vi "LAb7_MSK1.vi"() -> ()   [LabVIEW 2019]
uses:
  <vilib>/addons/Modulation/Digital/General/MT Generate Bits (Galois, PN Order).vi
  <vilib>/addons/Modulation/Analog/support/mod_Set Error Source.vi
  <vilib>/addons/Modulation/Digital/Support/Common/Validators/mod_Generate Bits Validate.vi
  <vilib>/addons/Modulation/Digital/Support/Common/Validators/mod_AWGN Validate.vi
  <vilib>/addons/Modulation/Digital/Impairments/subVIs/mod_createSeeds.vi
  <vilib>/addons/Modulation/Digital/Support/Common/Validators/mod_Validate Samples Per Symbol.vi
  <vilib>/addons/Modulation/Analog/support/Validators/mod_Validate Complex Waveform.vi
  <vilib>/addons/Modulation/Analog/support/Validators/mod_WFErrorHandler.vi
  <vilib>/addons/Modulation/Digital/General/subVIs/mod_Generate Bits PN Sequence.vi
  <vilib>/addons/Modulation/Digital/Support/Common/Validators/mod_Generate Filter Coefficients Validate.vi
  <vilib>/addons/Modulation/Digital/General/subVIs/mod_Generate Filter Coefficients.vi
  <vilib>/addons/Modulation/Digital/General/MT Generate MSK System Parameters.vi
  <vilib>/addons/Modulation/Digital/General/MT Map Bits to MSK symbols.vi
  <vilib>/addons/Modulation/Digital/General/MT Apply Pulse Shaping Filter (MSK).vi
  <vilib>/Analysis/1siggen.llb/Gaussian White Noise (obs 90).vi
  <vilib>/addons/Modulation/Analog/MT Upconvert Baseband (Real).vi
  <vilib>/express/express analysis/Spectral/Block/exnSpectralBlock spectral measurements RMS poly.vi
  <vilib>/express/express analysis/Spectral/Block/exnSpectralBlock spectral measurements RMS DDT.vi
  <vilib>/addons/Modulation/Digital/General/MT Apply Matched Filter (MSK).vi
  <vilib>/addons/Modulation/Digital/General/MT Align To Ideal Symbols (MSK).vi
  <vilib>/addons/Modulation/Digital/General/MT Map MSK Symbols to Bits.vi
  <vilib>/addons/Modulation/Digital/Demodulation/MT Calculate BER After Trigger (Fibonacci PN Sequence).vi
  <vilib>/express/express analysis/Spectral/XNode/ExpressSpectralMeasurementsBlockNode.xnode
  <vilib>/addons/Modulation/niDMT.lvlib
  <vilib>/addons/Modulation/niAMT.lvlib
panel:
  in  "Differential Encoding":u16(ring)=1 items=["disable", "enable"]
  in  "Pulse Shaping Filter":u16(ring) items=["none", "Raised Cosine", "Root Raised Cos", "Gaussian"]
  out "Constellation Graph":T1(graph)
  out "Recovered Message Bits":i8[](array[numeric])
  in  "Eb/N0 (dB)":dbl=10.0 format="%.2f"
  in  "autoscale":bool
  out "BER":dbl format="%.4f"
  out "error out":errorcluster
  out "Spectrum(FFT)":dynamicdata(graph)
  in  "stop":bool
  in  "Reset":bool=TRUE
  in  "Symbol Rate(HZ)":dbl=10.0 format="%.2p"
  in  "MSK Symbols":i32
  # "MSK"
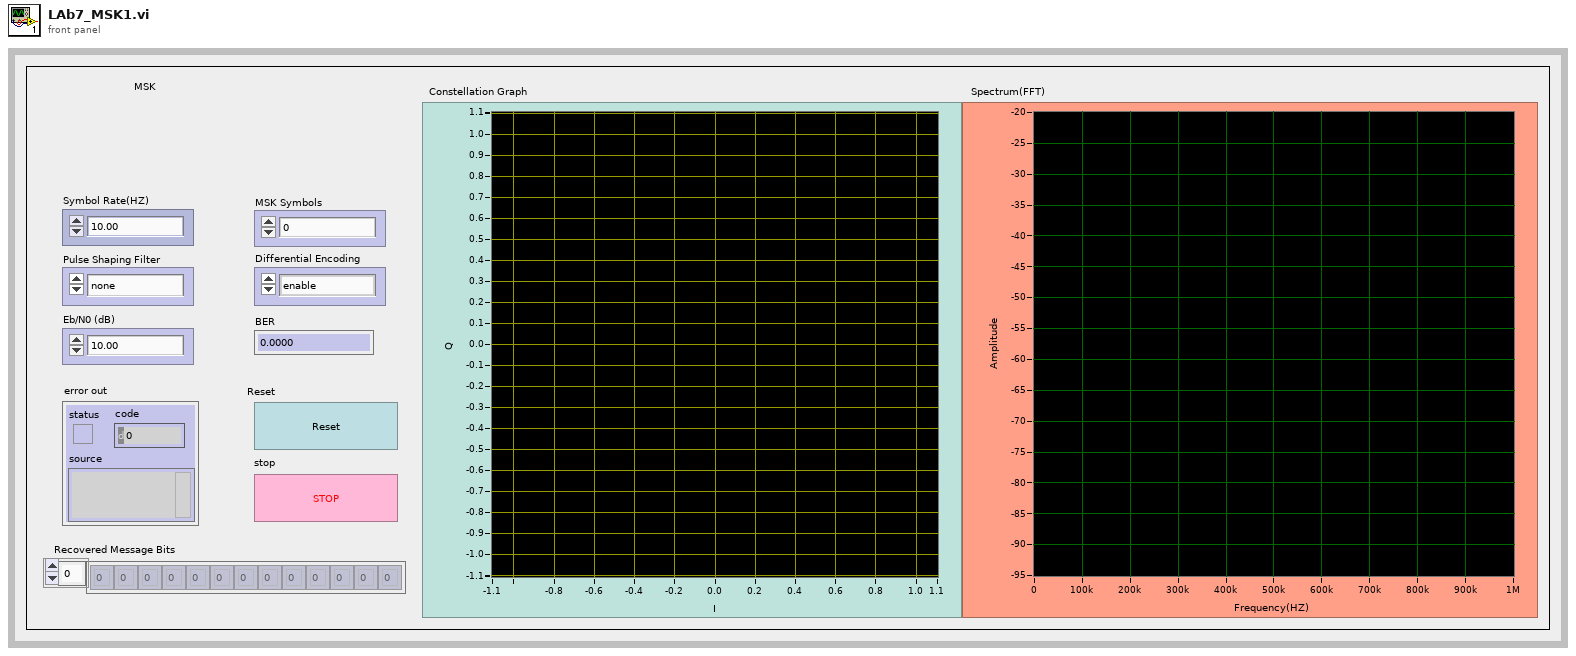
[diagram p1: front panel]
types:
  T1 = cluster{"Decimated Array":dbl[], "Decimated Array":dbl[]}[]
  T2 = enum16{"FSK", "PSK", "QAM", "MSK", "PAM", "ASK", "CPM"}
  T3 = cluster{"averaging mode":u16, "weighting mode":u16, "number of averages":u32}
  T4 = cluster{"dB On (F)":bool, "unwrap phase (F)":bool, "convert to degree (F)":bool}
  T5 = cluster{"differential encoding enable":enum16{"disable", "enable"}, "samples per symbol (16)":i32}
  T6 = typedef "niAMT.lvlib/Complex Data Waveform.ctl" = cluster{"t0":dbl, "dt":dbl, "Y":cdb[]}
  T7 = cluster{"constellation":dbl[], "oversampled data":dbl[]}[]
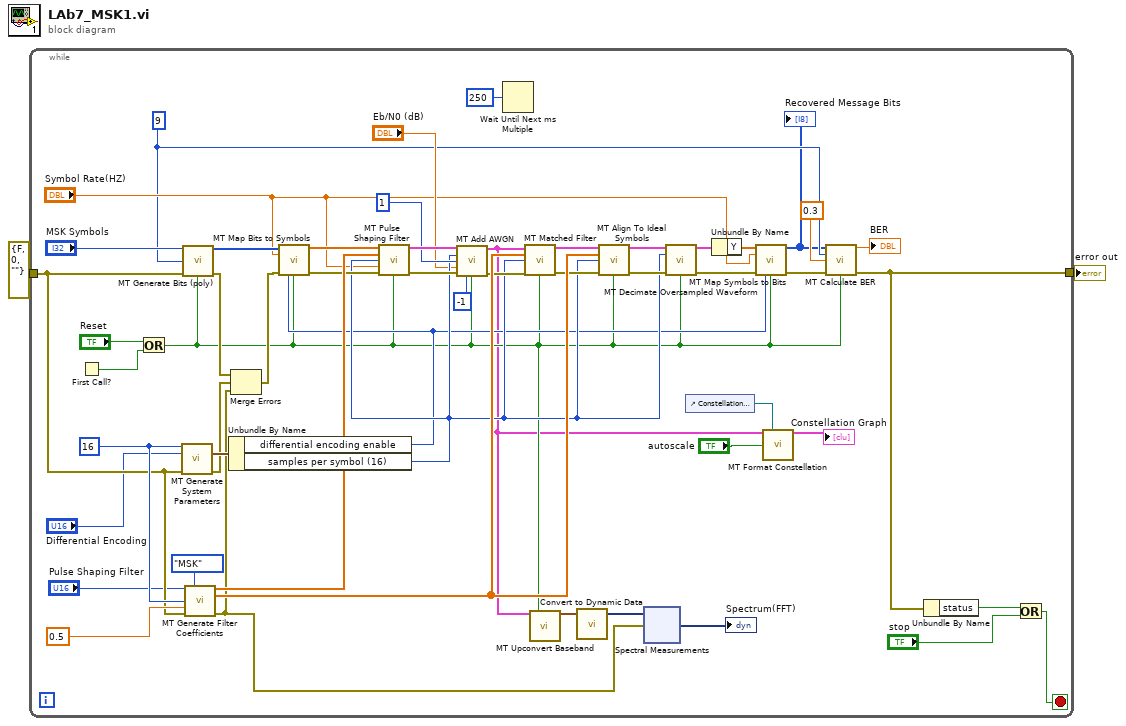
[diagram p0: block diagram]
diagram:
  n1 = while {
    tunnel: errorcluster {"status"=FALSE, "code"=0, "source"=""} ("error in (no error)") -> [w46]
    tunnel: [w14] -> w1
    stop <- w54 stop-if-true
    w48 = 16
    w8 = 9 ("samples per symbol (16)")
    n2 = First Call?() -> (First Call?: T/F=w18:bool)
    n3 = Or(x="Reset", y=w18) -> (x .or. y?=w19:bool)
    n4 = call-poly <vilib>:"MT Generate System Parameters.vi"("samples per symbol (16)"=w48, "differential encoding enable"="Differential Encoding", "error in (no error)"=w46) -> ("MSK system parameters"=w45:T5, "error out"=w24:errorcluster)  [unwired: 10 in, 1 out]
    n5 = call-poly <vilib>:"MT Generate Bits (poly).vi"("total bits (128)"="MSK Symbols", "PN sequence order (9)"=w8, "error in (no error)"=w46, "reset? (T)"=w19) -> ("output bit stream"=w44:i8[], "error out"=w26:errorcluster)  [unwired: 9 in, 1 out]
    n6 = call <vilib>:"MT Generate Filter Coefficients.vi"("pulse shaping filter (none)"="Pulse Shaping Filter", "modulation type"=T2."MSK", "matched samples per symbol (16)"=w48, "filter parameter"=0.5, "error in (no error)"=w46) -> ("pulse shaping filter coefficients"=w36:dbl[], "matched filter coefficients"=w35:dbl[], "error out"=w20:errorcluster)  [unwired: 8 in]
    n7 = Unbundle By Name(w45) -> ("differential encoding enable"=w27:enum16{"disable", "enable"}, "samples per symbol (16)"=w28:i32)
    n8 = Merge Errors(w26, w24, w20) -> (w25:errorcluster)
    n9 = call-poly <vilib>:"MT Map Bits to Symbols.vi"("input bit stream"=w44, "symbol rate, Hz"="Symbol Rate(HZ)", "error in (no error)"=w25, "differential encoding enable"=w27, "reset? (T)"=w19) -> ("symbols"=w43:dbl[], "error out"=w34:errorcluster)  [unwired: 9 in]
    n10 = call-poly <vilib>:"MT Pulse Shaping Filter.vi"("symbols"=w43, "pulse shaping filter coefficients"=w36, "samples per symbol (16)"=w28, "symbol rate (Hz)"="Symbol Rate(HZ)", "error in (no error)"=w34, "reset? (T)"=w19) -> ("output complex waveform"=w42:T6, "error out"=w33:errorcluster)  [unwired: 8 in]
    n11 = call <vilib>:"MT Add AWGN.vi"("input complex waveform"=w42, "samples per symbol (16)"=w28, "bits per symbol (1)"=1, "Eb/N0 (10 dB)"="Eb/N0 (dB)", "error in (no error)"=w33, "seed in (0xFFFFFFFF)"=-1, "reset? (T)"=w19) -> ("output complex waveform"=w12:T6, "error out"=w32:errorcluster)  [unwired: 6 in, 1 out]
    n12 = Wait Until Next ms Multiple(millisecond multiple=u32 250) -> ()  [unwired: 1 out]
    n13 = call-poly <vilib>:"MT Matched Filter.vi"("input complex waveform"=w12, "matched filter coefficients"=w35, "samples per symbol (16)"=w28, "error in (no error)"=w32, "reset? (T)"=w19) -> ("output phase waveform"=w40:cluster{"t0":dbl, "dt":dbl, "Y":dbl[]}, "error out"=w31:errorcluster)  [unwired: 9 in]
    n14 = call-poly <vilib>:"MT Upconvert Baseband.vi"("baseband waveform (complex)"=w12, "reset? (F)"=w19) -> ("passband waveform"=w21:waveform(dbl))  [unwired: 12 in, 1 out]
    n15 = call "Convert to Dynamic Data"("Waveform"=w21) -> ("Dynamic Data Type"=w22:dynamicdata)  [unwired: 3 in]
    n16 = call-poly <vilib>:"MT Align To Ideal Symbols.vi"("input phase waveform"=w40, "matched filter coefficients"=w35, "samples per symbol (16)"=w28, "error in (no error)"=w31, "reset? (T)"=w19) -> ("output phase waveform"=w39:cluster{"t0":dbl, "dt":dbl, "Y":dbl[]}, "error out"=w30:errorcluster)  [unwired: 8 in, 1 out]
    n17 = xnode "Spectral Measurements"("Signals"=w22, "error in (no error)"=w20) -> ("FFT - (RMS)"=→"Spectrum(FFT)":dynamicdata)  [unwired: 2 out]
    n18 = call <vilib>:"MT Decimate Oversampled Waveform.vi"("input complex waveform"=w39, "decimation factor"=w28, "error in (no error)"=w30, "reset? (T)"=w19) -> ("output complex waveform"=w38:T6, "error out"=w41:errorcluster)  [unwired: 10 in]
    n19 = control-ref of="Constellation Graph"() -> (w52:refnum<vi>)
    n20 = Unbundle By Name(w38) -> ("Y"=w37:cdb[])
    n21 = call-poly <vilib>:"MT Map Symbols to Bits.vi"("symbols"=w37, "symbol rate"="Symbol Rate(HZ)", "error in (no error)"=w41, "differential encoding enable"=w27, "reset? (T)"=w19) -> ("output bit stream"=w7:i8[], "error out"=w16:errorcluster)  [unwired: 9 in]
    "Recovered Message Bits" <- w7
    n22 = call <vilib>:"MT Format Constellation.vi"("waveform"=w12, "constellation reference"=w52, "autoscale"="autoscale") -> ("constellation graph"=→"Constellation Graph":T7)  [unwired: 2 in, 10 out]
    n23 = call-poly <vilib>:"MT Calculate BER.vi"("input bit stream"=w7, "PN sequence order (9)"=w8, "BER trigger threshold (0.1)"=0.3, "error in (no error)"=w16, "reset? (T)"=w19) -> ("BER"=→"BER":dbl, "error out"=w14:errorcluster)  [unwired: 6 in, 3 out]
    n24 = Unbundle By Name(w14) -> ("status"=w17:bool)
    n25 = Or(x=w17, y="stop") -> (x .or. y?=w54:bool)
  }
  "error out" <- w1
